vi "Extract subclasses from Magnet device.vi"(9 "Data In":string, 10 "Class":string, 11 "Aux Device Settings in":T1={"Manufacturing"={"Hardware Version"="", "Firmware Version"="", "Serial Number"=""}, "Nickname"="", "Bipolar Output"="", "String"="SERS", "Current Limit"=0.0, "AtoB"=0.0, "Inductance"=0.0, "Switch Present"="", "Swh Htr Current"=0.0, "SW VLIM"=0.0, "V Trans Time"=0.0, "Magnet PSU Signals"={"Voltage"=0.0, "Current"=0.0, "Current Rate"=0.0, "Field"=0.0, "Field Rate"=0.0, "Persistant Current"=0.0, "Persistant Field"=0.0, "Target Current"=0.0, "Target Field"=0.0, "Target Current Rate"=0.0, "Target Field Rate"=0.0, "Switch Heater Status (SWHT)"="", "Switch Heater Status (SWHN)"=""}, "PSU Action"="SERS", "Status"="", "Level Limit"=0.0, "Temperature Limit"=0.0} {"Temperature Limit" format="%#.1f"; "Level Limit" format="%#.1f"; "V Trans Time" format="%#.1f"; "SW VLIM" format="%#.1f"; "Swh Htr Current" format="%#.1f"; "Inductance" format="%#.1f"; "AtoB" format="%#.1f"; "Current Limit" format="%#.1f"}) -> (1 "Data out":string, 3 "Aux Device Settings out":T1={"Manufacturing"={"Hardware Version"="", "Firmware Version"="", "Serial Number"=""}, "Nickname"="", "Bipolar Output"="", "String"="SERS", "Current Limit"=0.0, "AtoB"=0.0, "Inductance"=0.0, "Switch Present"="", "Swh Htr Current"=0.0, "SW VLIM"=0.0, "V Trans Time"=0.0, "Magnet PSU Signals"={"Voltage"=0.0, "Current"=0.0, "Current Rate"=0.0, "Field"=0.0, "Field Rate"=0.0, "Persistant Current"=0.0, "Persistant Field"=0.0, "Target Current"=0.0, "Target Field"=0.0, "Target Current Rate"=0.0, "Target Field Rate"=0.0, "Switch Heater Status (SWHT)"="", "Switch Heater Status (SWHN)"=""}, "PSU Action"="SERS", "Status"="", "Level Limit"=0.0, "Temperature Limit"=0.0} {"Temperature Limit" format="%#.1f"; "Level Limit" format="%#.1f"; "V Trans Time" format="%#.1f"; "SW VLIM" format="%#.1f"; "Swh Htr Current" format="%#.1f"; "Inductance" format="%#.1f"; "AtoB" format="%#.1f"; "Current Limit" format="%#.1f"})   [LabVIEW 2015, in "Mercury iXX.lvlib" / "Magnet.lvlib"]
uses:
  Magnet.lvlib
  Controls/Device (Read).ctl
  Controls/Manufacturing Data.ctl
  Controls/Signals (Read).ctl
  Mercury iXX.lvlib
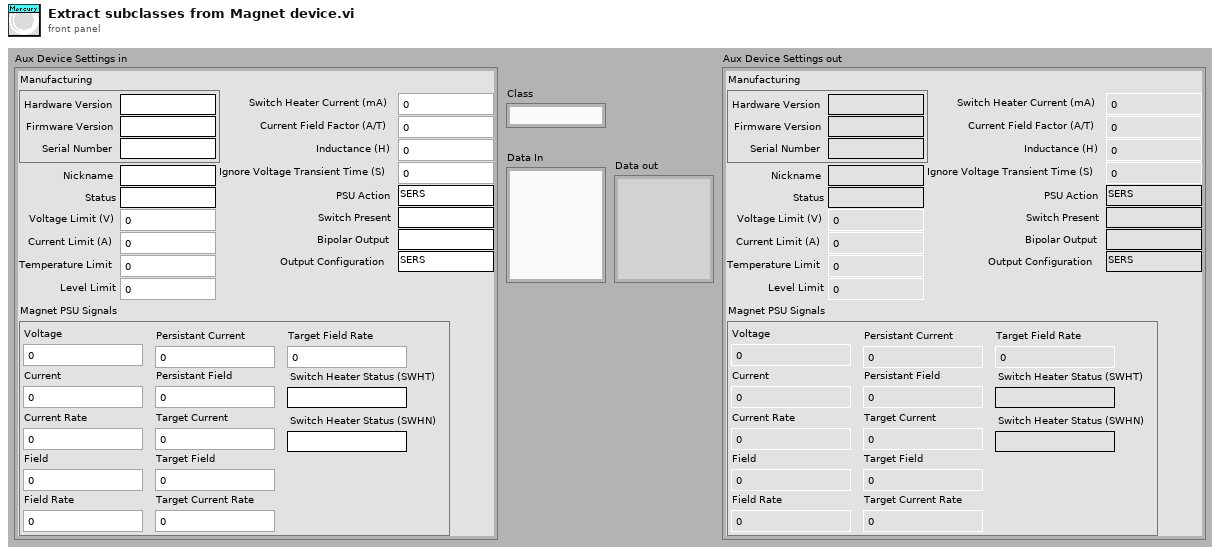
[diagram p1: front panel]
types:
  T1 = typedef "Mercury iXX.lvlib/Magnet.lvlib/Device (Read).ctl" = cluster{"Manufacturing":T2, "Nickname":string, "Bipolar Output":string, "String":string, "Current Limit":dbl, "AtoB":dbl, "Inductance":dbl, "Switch Present":string, "Swh Htr Current":dbl, "SW VLIM":dbl, "V Trans Time":dbl, "Magnet PSU Signals":T3, "PSU Action":string, "Status":string, "Level Limit":dbl, "Temperature Limit":dbl}
  T2 = typedef "Mercury iXX.lvlib/Manufacturing Data.ctl" = cluster{"Hardware Version":string, "Firmware Version":string, "Serial Number":string}
  T3 = typedef "Mercury iXX.lvlib/Magnet.lvlib/Signals (Read).ctl" = cluster{"Voltage":dbl, "Current":dbl, "Current Rate":dbl, "Field":dbl, "Field Rate":dbl, "Persistant Current":dbl, "Persistant Field":dbl, "Target Current":dbl, "Target Field":dbl, "Target Current Rate":dbl, "Target Field Rate":dbl, "Switch Heater Status (SWHT)":string, "Switch Heater Status (SWHN)":string}
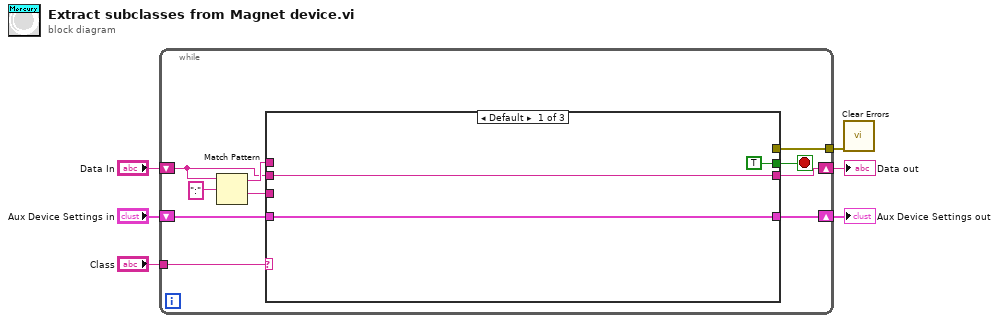
[diagram p0: block diagram]
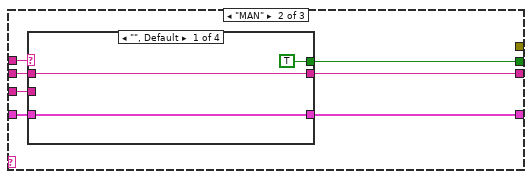
[diagram p2: hidden frame]
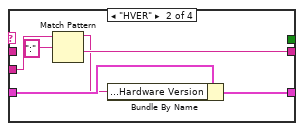
[diagram p3: hidden frame]
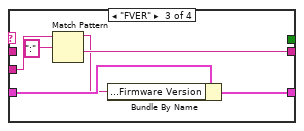
[diagram p4: hidden frame]
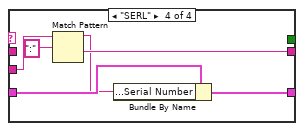
[diagram p5: hidden frame]
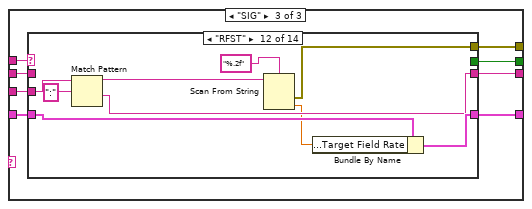
[diagram p6: hidden frame]
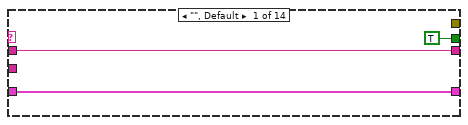
[diagram p7: hidden frame]
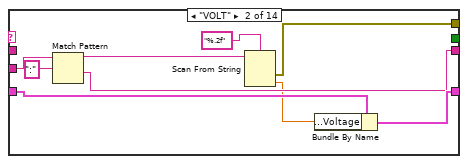
[diagram p8: hidden frame]
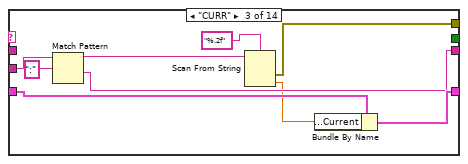
[diagram p9: hidden frame]
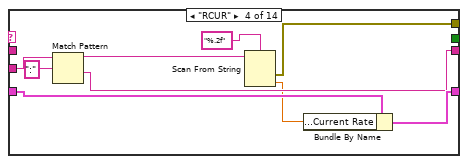
[diagram p10: hidden frame]
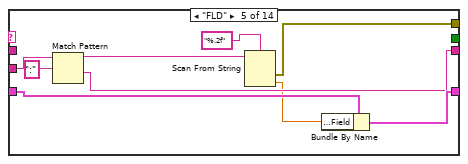
[diagram p11: hidden frame]
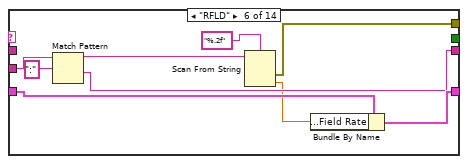
[diagram p12: hidden frame]
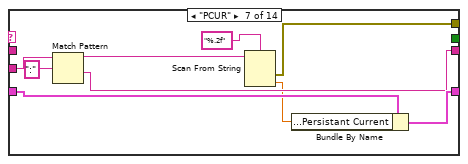
[diagram p13: hidden frame]
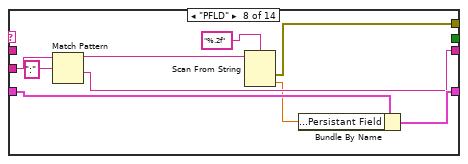
[diagram p14: hidden frame]
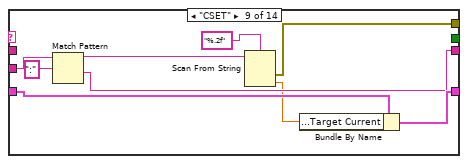
[diagram p15: hidden frame]
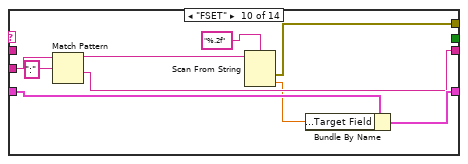
[diagram p16: hidden frame]
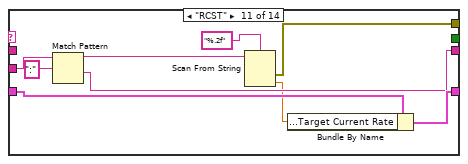
[diagram p17: hidden frame]
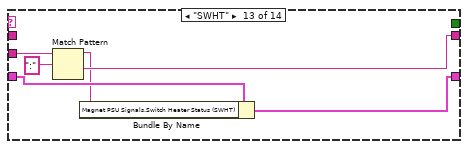
[diagram p18: hidden frame]
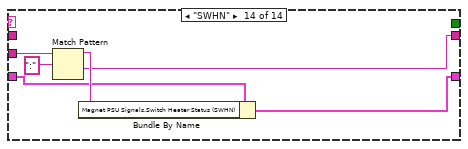
[diagram p19: hidden frame]
diagram:
  n1 = while {
    tunnel: "Class" -> [w15]
    shift-right: [w9] -> w5
    shift-left: "Data In" -> [w11]
    shift-right: [w10] -> w4
    shift-left: "Aux Device Settings in" -> [w12]
    tunnel: [w7] -> w1
    stop <- w8 stop-if-true
    n2 = Match Pattern(string=w11, regular expression=":") -> (before substring=w14:string, after substring=w13:string)  [unwired: 3 out]
    n3 = case shown="Default" w15 {
      tunnel: w12 -> [w19 w26 w55]
      tunnel: [w19 w25 w50] -> w10
      tunnel: w13 -> [_ w24 w53]
      tunnel: [w18 w23 w49] -> w9
      tunnel: w14 -> [_ w22 w54]
      tunnel: w11 -> [w18 w21 w52]
      tunnel: [TRUE w20 w51] -> w8
      tunnel: [_ _ w48] -> w7
      frame Default {
      }
      frame "MAN" {
        n4 = case shown="\"\", Default" w22 {
          tunnel: w26 -> [w29 w35 w41 w47]
          tunnel: [w29 w34 w40 w46] -> w25
          tunnel: w24 -> [_ w33 w39 w45]
          tunnel: [w28 w32 w38 w44] -> w23
          tunnel: w21 -> [w28 _ _ _]
          tunnel: [TRUE _ _ _] -> w20
          frame "", Default {
          }
          frame "HVER" {
            n5 = Match Pattern(string=w33, regular expression=":") -> (before substring=w30:string, after substring=w32:string)  [unwired: 3 out]
            n6 = Bundle By Name(cluster=w35, "Manufacturing.Hardware Version"=w30) -> (w34:T1)
          }
          frame "FVER" {
            n7 = Match Pattern(string=w39, regular expression=":") -> (before substring=w36:string, after substring=w38:string)  [unwired: 3 out]
            n8 = Bundle By Name(cluster=w41, "Manufacturing.Firmware Version"=w36) -> (w40:T1)
          }
          frame "SERL" {
            n9 = Match Pattern(string=w45, regular expression=":") -> (before substring=w42:string, after substring=w44:string)  [unwired: 3 out]
            n10 = Bundle By Name(cluster=w47, "Manufacturing.Serial Number"=w42) -> (w46:T1)
          }
        }
      }
      frame "SIG" {
        n11 = case shown="\"RFST\"" w54 {
          tunnel: w55 -> [w58 w67 w76 w85 w94 w103 w112 w121 w130 w139 w148 w157 w163 w167]
          tunnel: [w58 w66 w75 w84 w93 w102 w111 w120 w129 w138 w147 w156 w162 w165] -> w50
          tunnel: w53 -> [_ w65 w74 w83 w92 w101 w110 w119 w128 w137 w146 w155 w161 w166]
          tunnel: [w57 w64 w73 w82 w91 w100 w109 w118 w127 w136 w145 w154 w160 w164] -> w49
          tunnel: w52 -> [w57 _ _ _ _ _ _ _ _ _ _ _ _ _]
          tunnel: [TRUE _ _ _ _ _ _ _ _ _ _ _ _ _] -> w51
          tunnel: [_ w59 w68 w77 w86 w95 w104 w113 w122 w131 w140 w149 _ _] -> w48
          frame "", Default {
          }
          frame "VOLT" {
            n12 = Match Pattern(string=w65, regular expression=":") -> (before substring=w62:string, after substring=w64:string)  [unwired: 3 out]
            n13 = Scan From String(format string="%.2f", input string=w62) -> (error out=w59:errorcluster, output 1=w61:dbl)  [unwired: 2 in, 3 out]
            n14 = Bundle By Name(cluster=w67, "Magnet PSU Signals.Voltage"=w61) -> (w66:T1)
          }
          frame "CURR" {
            n15 = Match Pattern(string=w74, regular expression=":") -> (before substring=w71:string, after substring=w73:string)  [unwired: 3 out]
            n16 = Scan From String(format string="%.2f", input string=w71) -> (error out=w68:errorcluster, output 1=w70:dbl)  [unwired: 2 in, 3 out]
            n17 = Bundle By Name(cluster=w76, "Magnet PSU Signals.Current"=w70) -> (w75:T1)
          }
          frame "RCUR" {
            n18 = Match Pattern(string=w83, regular expression=":") -> (before substring=w80:string, after substring=w82:string)  [unwired: 3 out]
            n19 = Scan From String(format string="%.2f", input string=w80) -> (error out=w77:errorcluster, output 1=w79:dbl)  [unwired: 2 in, 3 out]
            n20 = Bundle By Name(cluster=w85, "Magnet PSU Signals.Current Rate"=w79) -> (w84:T1)
          }
          frame "FLD" {
            n21 = Match Pattern(string=w92, regular expression=":") -> (before substring=w89:string, after substring=w91:string)  [unwired: 3 out]
            n22 = Scan From String(format string="%.2f", input string=w89) -> (error out=w86:errorcluster, output 1=w88:dbl)  [unwired: 2 in, 3 out]
            n23 = Bundle By Name(cluster=w94, "Magnet PSU Signals.Field"=w88) -> (w93:T1)
          }
          frame "RFLD" {
            n24 = Match Pattern(string=w101, regular expression=":") -> (before substring=w98:string, after substring=w100:string)  [unwired: 3 out]
            n25 = Scan From String(format string="%.2f", input string=w98) -> (error out=w95:errorcluster, output 1=w97:dbl)  [unwired: 2 in, 3 out]
            n26 = Bundle By Name(cluster=w103, "Magnet PSU Signals.Field Rate"=w97) -> (w102:T1)
          }
          frame "PCUR" {
            n27 = Match Pattern(string=w110, regular expression=":") -> (before substring=w107:string, after substring=w109:string)  [unwired: 3 out]
            n28 = Scan From String(format string="%.2f", input string=w107) -> (error out=w104:errorcluster, output 1=w106:dbl)  [unwired: 2 in, 3 out]
            n29 = Bundle By Name(cluster=w112, "Magnet PSU Signals.Persistant Current"=w106) -> (w111:T1)
          }
          frame "PFLD" {
            n30 = Match Pattern(string=w119, regular expression=":") -> (before substring=w116:string, after substring=w118:string)  [unwired: 3 out]
            n31 = Scan From String(format string="%.2f", input string=w116) -> (error out=w113:errorcluster, output 1=w115:dbl)  [unwired: 2 in, 3 out]
            n32 = Bundle By Name(cluster=w121, "Magnet PSU Signals.Persistant Field"=w115) -> (w120:T1)
          }
          frame "CSET" {
            n33 = Match Pattern(string=w128, regular expression=":") -> (before substring=w125:string, after substring=w127:string)  [unwired: 3 out]
            n34 = Scan From String(format string="%.2f", input string=w125) -> (error out=w122:errorcluster, output 1=w124:dbl)  [unwired: 2 in, 3 out]
            n35 = Bundle By Name(cluster=w130, "Magnet PSU Signals.Target Current"=w124) -> (w129:T1)
          }
          frame "FSET" {
            n36 = Match Pattern(string=w137, regular expression=":") -> (before substring=w134:string, after substring=w136:string)  [unwired: 3 out]
            n37 = Scan From String(format string="%.2f", input string=w134) -> (error out=w131:errorcluster, output 1=w133:dbl)  [unwired: 2 in, 3 out]
            n38 = Bundle By Name(cluster=w139, "Magnet PSU Signals.Target Field"=w133) -> (w138:T1)
          }
          frame "RCST" {
            n39 = Match Pattern(string=w146, regular expression=":") -> (before substring=w143:string, after substring=w145:string)  [unwired: 3 out]
            n40 = Scan From String(format string="%.2f", input string=w143) -> (error out=w140:errorcluster, output 1=w142:dbl)  [unwired: 2 in, 3 out]
            n41 = Bundle By Name(cluster=w148, "Magnet PSU Signals.Target Current Rate"=w142) -> (w147:T1)
          }
          frame "RFST" {
            n42 = Match Pattern(string=w155, regular expression=":") -> (before substring=w152:string, after substring=w154:string)  [unwired: 3 out]
            n43 = Scan From String(format string="%.2f", input string=w152) -> (error out=w149:errorcluster, output 1=w151:dbl)  [unwired: 2 in, 3 out]
            n44 = Bundle By Name(cluster=w157, "Magnet PSU Signals.Target Field Rate"=w151) -> (w156:T1)
          }
          frame "SWHT" {
            n45 = Match Pattern(string=w161, regular expression=":") -> (before substring=w158:string, after substring=w160:string)  [unwired: 3 out]
            n46 = Bundle By Name(cluster=w163, "Magnet PSU Signals.Switch Heater Status (SWHT)"=w158) -> (w162:T1)
          }
          frame "SWHN" {
            n47 = Match Pattern(string=w166, regular expression=":") -> (before substring=w168:string, after substring=w164:string)  [unwired: 3 out]
            n48 = Bundle By Name(cluster=w167, "Magnet PSU Signals.Switch Heater Status (SWHN)"=w168) -> (w165:T1)
          }
        }
      }
    }
  }
  "Data out" <- w5
  "Aux Device Settings out" <- w4
  n49 = call <vilib>:"Clear Errors.vi"("error in (no error)"=w1) -> ()  [unwired: 1 in, 6 out]
